vi "PointMap_Destroy.vi"(8 "error in (no error)":errorcluster, 10 "Name":string) -> (0 "error out":errorcluster)   [LabVIEW 2017, in "PointValueMap.lvlib"]
doc: "Deletes a point value map from memory."
uses:
  <vilib>/addons/PointValueMap/PointValueMap.lvlib
  <vilib>/addons/PointValueMap/controls/PointMapOperations.ctl
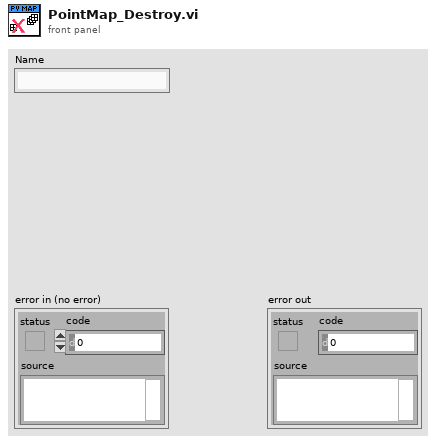
[diagram p1: front panel]
types:
  T1 = typedef "PointValueMap.lvlib/PointMapOperations.ctl" = enum16{"Initialize", "Create Map", "Update Map", "Get Map", "Get All Maps", "Destroy Map", "Destroy All Maps"}
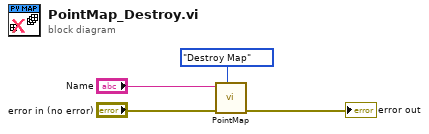
[diagram p0: block diagram]
diagram:
  n1 = call <vilib>:"PointMap.vi"("Operation"=PointMapOperations."Destroy Map", "error in (no error)"="error in (no error)", "Name"="Name") -> ("error out"=→"error out":errorcluster)  [unwired: 4 in, 4 out]
